vi "CLD 2 Elapsed Time Express FGV Solution.vi"(7 "Express Timer FGV Enum":enum16{"Reset", "Read Status", "Set Auto Reset"}(ring), 8 "error in (no error)":errorcluster, 9 "Auto Reset (F)":bool, 11 "Time Target (s)":dbl=7.0) -> (0 "error out":errorcluster, 2 "Elapsed Time (s)":dbl, 3 "Time Has Elapsed":bool)   [LabVIEW 2020]
doc: "CLD 2 Exercise"
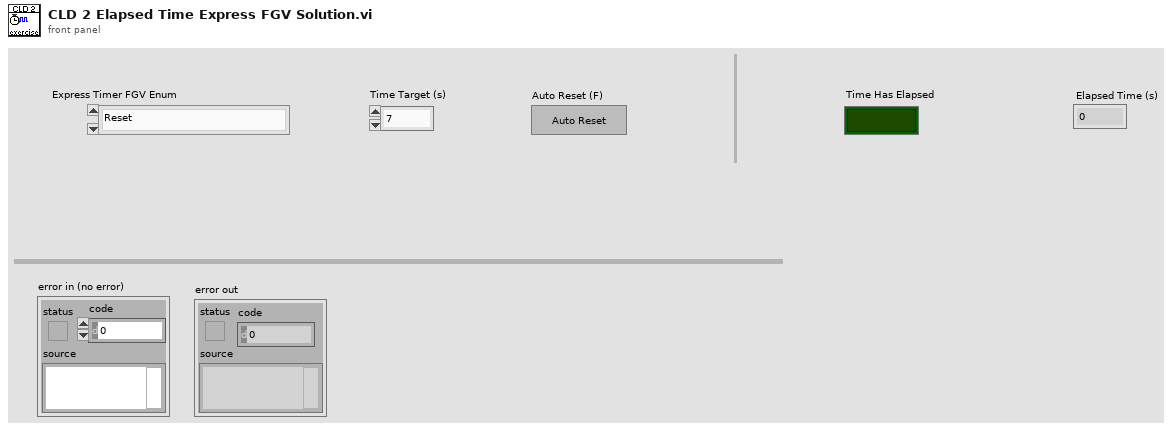
[diagram p1: front panel]
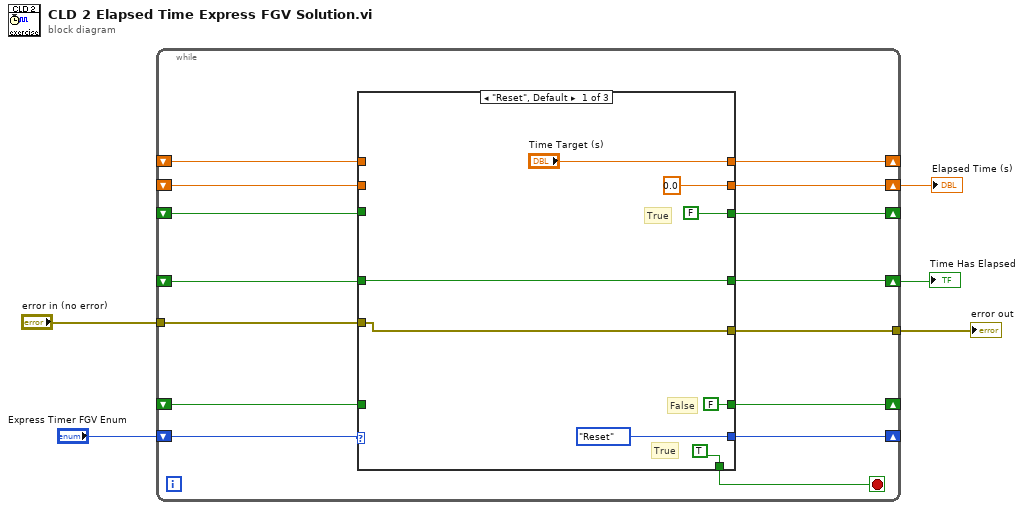
[diagram p0: block diagram]
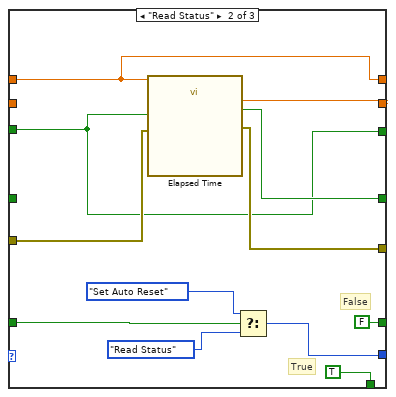
[diagram p2: hidden frame]
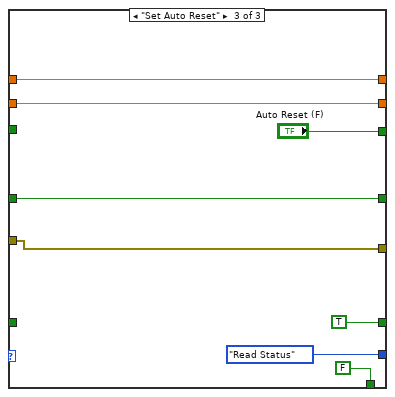
[diagram p3: hidden frame]
diagram:
  n1 = while {
    shift-right: [w20] -> _
    shift-left: _ -> [w16]
    shift-right: [w18] -> _
    shift-left: _ -> [w17]
    tunnel: "error in (no error)" -> [w15]
    tunnel: [w14] -> w3
    shift-right: [w13] -> w2
    shift-left: _ -> [w12]
    shift-right: [w19] -> w5
    shift-left: _ -> [w11]
    shift-right: [w9] -> _
    shift-left: "Express Timer FGV Enum" -> [w10]
    shift-right: [w7] -> _
    shift-left: _ -> [w6]
    stop <- w8 stop-if-true
    n2 = case shown="\"Reset\", Default" w10 {
      tunnel: ["Time Target (s)" w29 w45] -> w20
      tunnel: w16 -> [_ w29 w45]
      tunnel: [0.0 ("Elapsed Time (s)") w40 w44] -> w19
      tunnel: [FALSE ("Auto Reset (F)") w36 "Auto Reset (F)"] -> w18
      tunnel: w17 -> [_ w36 _]
      tunnel: w15 -> [w25 w39 w48]
      tunnel: [w25 w38 w48] -> w14
      tunnel: [w24 w37 w46] -> w13
      tunnel: w12 -> [w24 _ w46]
      tunnel: w11 -> [_ _ w44]
      tunnel: [enum16{"Reset", "Read Status", "Set Auto Reset"}."Reset" ("Express Timer FGV Enum") w31 enum16{"Reset", "Read Status", "Set Auto Reset"}."Read Status" ("Express Timer FGV Enum")] -> w9
      tunnel: [TRUE TRUE FALSE] -> w8
      tunnel: [FALSE FALSE TRUE] -> w7
      tunnel: w6 -> [_ w34 _]
      frame "Reset", Default {
        # "False"
        # "True"
        # "True"
      }
      frame "Read Status" {
        # "True"
        # "False"
        n3 = call "Elapsed Time"("Time Target (s)"=w29, "Auto Reset"=w36, "error in (no error)"=w39) -> ("Elapsed Time (s)"=w40:dbl, "Time has Elapsed"=w37:bool, "error out"=w38:errorcluster)  [unwired: 9 in, 5 out]
        n4 = Select(t=enum16{"Reset", "Read Status", "Set Auto Reset"}."Set Auto Reset" ("Express Timer FGV Enum"), s=w34, f=enum16{"Reset", "Read Status", "Set Auto Reset"}."Read Status" ("Express Timer FGV Enum")) -> (s? t:f=w31:enum16{"Reset", "Read Status", "Set Auto Reset"})
      }
      frame "Set Auto Reset" {
      }
    }
  }
  "error out" <- w3
  "Elapsed Time (s)" <- w5
  "Time Has Elapsed" <- w2
